vi "GT Get Di Reverse Count.vi"(6 "count":i16, 7 "pReverseCount":u32[](array[numeric]), 8 "error in (no error)":errorcluster caption="错误输入（无错误）", 9 "diIndex":i16, 10 "diType":i16, 11 "cardNum":i16) -> (0 "error out":errorcluster caption="错误输出", 3 "function return":i16, 5 "pReverseCount out":u32[](array[numeric]))   [LabVIEW 2020, in "gts.lvlib"]
doc: "GT_API GT_GetDiReverseCount(short cardNum,short diType,short diIndex,unsigned long *pReverseCount,short count=1);"
uses:
  gts.lvlib
  dll/32bit/multi_card/gts.dll
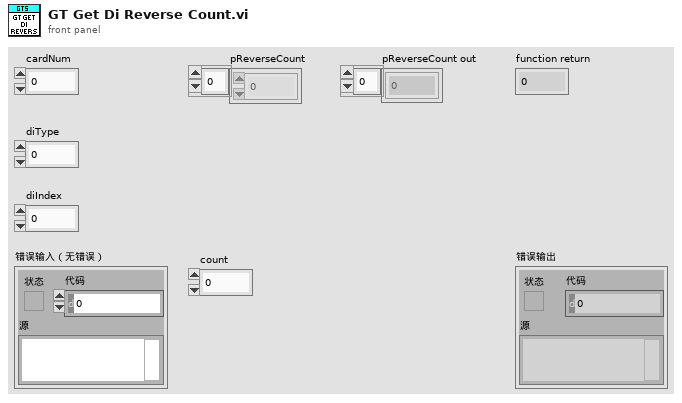
[diagram p1: front panel]
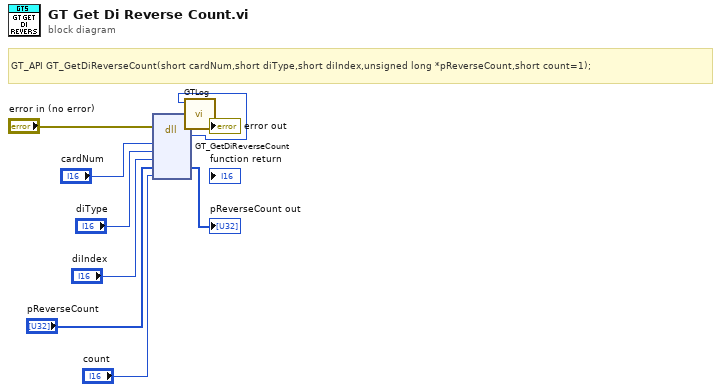
[diagram p0: block diagram]
diagram:
  # "GT_API GT_GetDiReverseCount(short cardNum,short diType,short diIndex,unsigned long *pReverseCount,short count=1);"
  n1 = dll-call lib="C:/1228/dll/32bit/multi_card/gts.dll" fn="GT_GetDiReverseCount"(error in="error in (no error)", "cardNum"="cardNum", "diType"="diType", "diIndex"="diIndex", "pReverseCount"="pReverseCount", "count"="count") -> (error out=w3:errorcluster, "返回类型"=w1:i16, "pReverseCount"=→"pReverseCount out":u32[])  [unwired: 6 in, 1 out]
  n2 = call "GTLog.vi"("error in (no error)"=w3, "Numeric"=w1) -> ("error out"=→"error out":errorcluster)  [unwired: 9 in]
